vi "async metadata time spec.vi"(8 "error in (no error)":errorcluster, 9 "frac_secs_out":dbl, 10 "full_secs_out":i64, 11 "h":u64) -> (0 "error out":errorcluster, 1 "frac_secs_out out":dbl, 2 "full_secs_out out":i64, 3 "h out":u64, 5 "function return":u32(ring))   [LabVIEW 2023, in "uhd.lvlib"]
doc: "UHD_API uhd_error uhd_async_metadata_time_spec(\n uhd_async_metadata_handle h, int64_t* full_secs_out, double* frac_secs_out);"
uses:
  <userlib>/uhd/uhd.lvlib
  <userlib>/uhd/uhd.dll
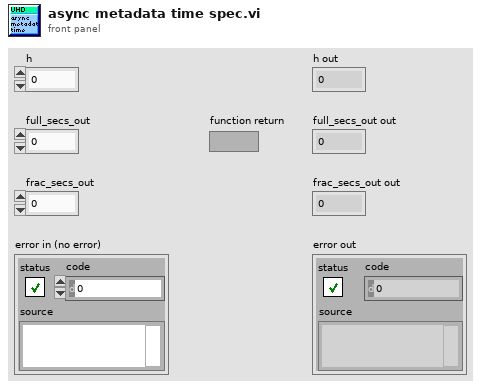
[diagram p1: front panel]
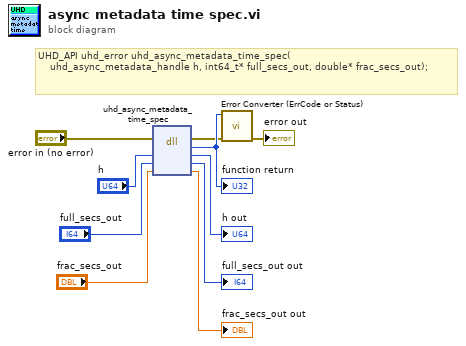
[diagram p0: block diagram]
diagram:
  # "UHD_API uhd_error uhd_async_metadata_time_spec(\n    uhd_async_metadata_handle h, int64_t* full_secs_out, double* frac_secs_out);"
  n1 = dll-call lib="C:/Program Files/National Instruments/LabVIEW 2023/user.lib/uhd/uhd.*" fn="uhd_async_metadata_time_spec"(error in="error in (no error)", "h"="h", "full_secs_out"="full_secs_out", "frac_secs_out"="frac_secs_out") -> (error out=w2:errorcluster, w10:u32, "h"=→"h out":u64, "full_secs_out"=→"full_secs_out out":i64, "frac_secs_out"=→"frac_secs_out out":dbl)  [unwired: 2 in, 1 out]
  "function return" <- w10
  n2 = call <userlib>:"Error Converter (ErrCode or Status).vi"("error in (no error)"=w2, "error code"=w10) -> ("error out"=→"error out":errorcluster)  [unwired: 9 in]
